vi "DeltaToWye.vi"() -> ()   [LabVIEW 2015]
panel:
  in  "aMod":dbl format="%#_13g"
  in  "bMod":dbl format="%#_13g"
  in  "cMod":dbl format="%#_13g"
  out "appended array":dbl[][](graph)
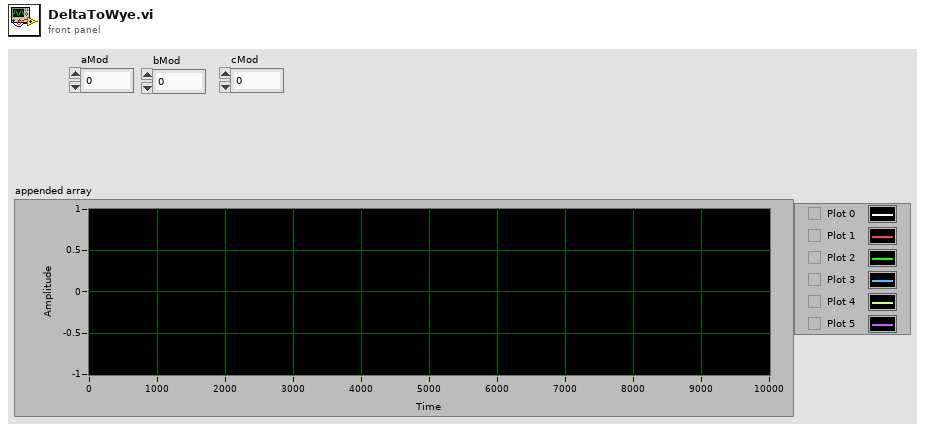
[diagram p1: front panel]
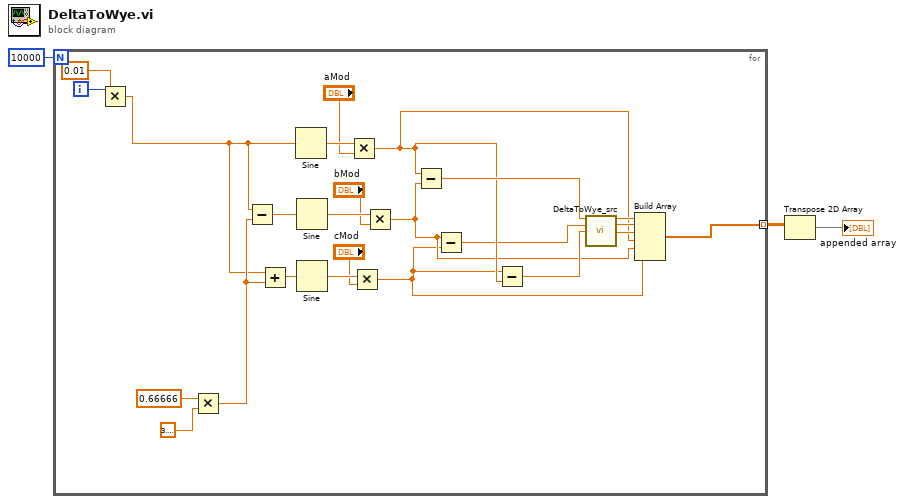
[diagram p0: block diagram]
diagram:
  n1 = for {
    N: 10000 -> [_]
    tunnel: [w15] -> w2 mode=indexing
    i -> [w22]
    n2 = Multiply(x=w22, y=0.01) -> (x*y=w16:dbl)
    n3 = Multiply(x=0.66666, y=3.141592653589793) -> (x*y=w23:dbl)
    n4 = Subtract(x=w16, y=w23) -> (x-y=w25:dbl)
    n5 = Add(x=w16, y=w23) -> (x+y=w24:dbl)
    n6 = Sine(x=w16) -> (sin(x)=w13:dbl)
    n7 = Sine(x=w25) -> (sin(x)=w11:dbl)
    n8 = Sine(x=w24) -> (sin(x)=w14:dbl)
    n9 = Multiply(x=w13, y="aMod") -> (x*y=w8:dbl)
    n10 = Multiply(x=w14, y="cMod") -> (x*y=w4:dbl)
    n11 = Multiply(x=w11, y="bMod") -> (x*y=w5:dbl)
    n12 = Subtract(x=w8, y=w5) -> (x-y=w20:dbl)
    n13 = Subtract(x=w5, y=w4) -> (x-y=w7:dbl)
    n14 = Subtract(x=w4, y=w8) -> (x-y=w6:dbl)
    n15 = call "DeltaToWye_src.vi"("AB"=w20, "BC"=w7, "CA"=w6) -> ("A"=w19:sgl, "B"=w18:sgl, "C"=w17:sgl)  [unwired: 10 in]
    n16 = Build Array(w19, w18, w17, w8, w5, w4) -> (w15:dbl[])
  }
  n17 = Transpose 2D Array(2D array=w2) -> (transposed array=→"appended array":dbl[][])
